vi "Array to csv string.vi"(11 "Array":string[](array[string])) -> (3 "spreadsheet string":string)   [LabVIEW 2018]
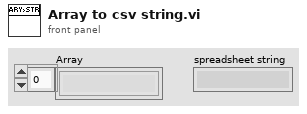
[diagram p1: front panel]
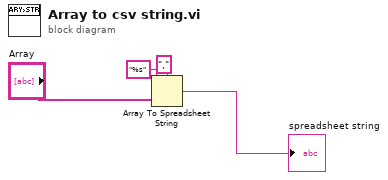
[diagram p0: block diagram]
diagram:
  n1 = Array To Spreadsheet String(delimiter (Tab)=",", array="Array", 3:"%s" ("format string")) -> (spreadsheet string=→"spreadsheet string":string)
